vi "Set Pump Phases Parameters 2 (SubVI).vi"(0 "Units":string, 1 "Target Time":dbl, 2 "error out 2":errorcluster, 4 "Inc/Dec time":dbl, 6 "Flow rate":dbl, 7 "Previous Flow rate":dbl, 8 "Direction":string(combo), 10 "Send":bool, 11 "VISA Pump resource name out 2":refnum<visa-resource-name>) -> (3 "VISA resource name out":refnum<visa-resource-name>, 5 "error out":errorcluster)   [LabVIEW 2020]
panel:
  in  "Valve error out 2":errorcluster
  in  "Valve Position":dbl
  in  "Valve VISA resource name":refnum<visa-resource-name>
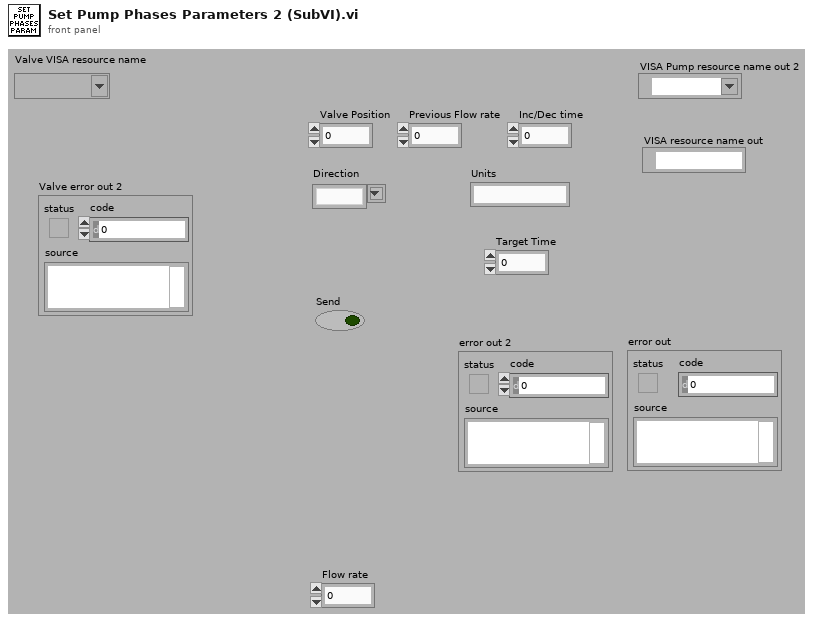
[diagram p1: front panel]
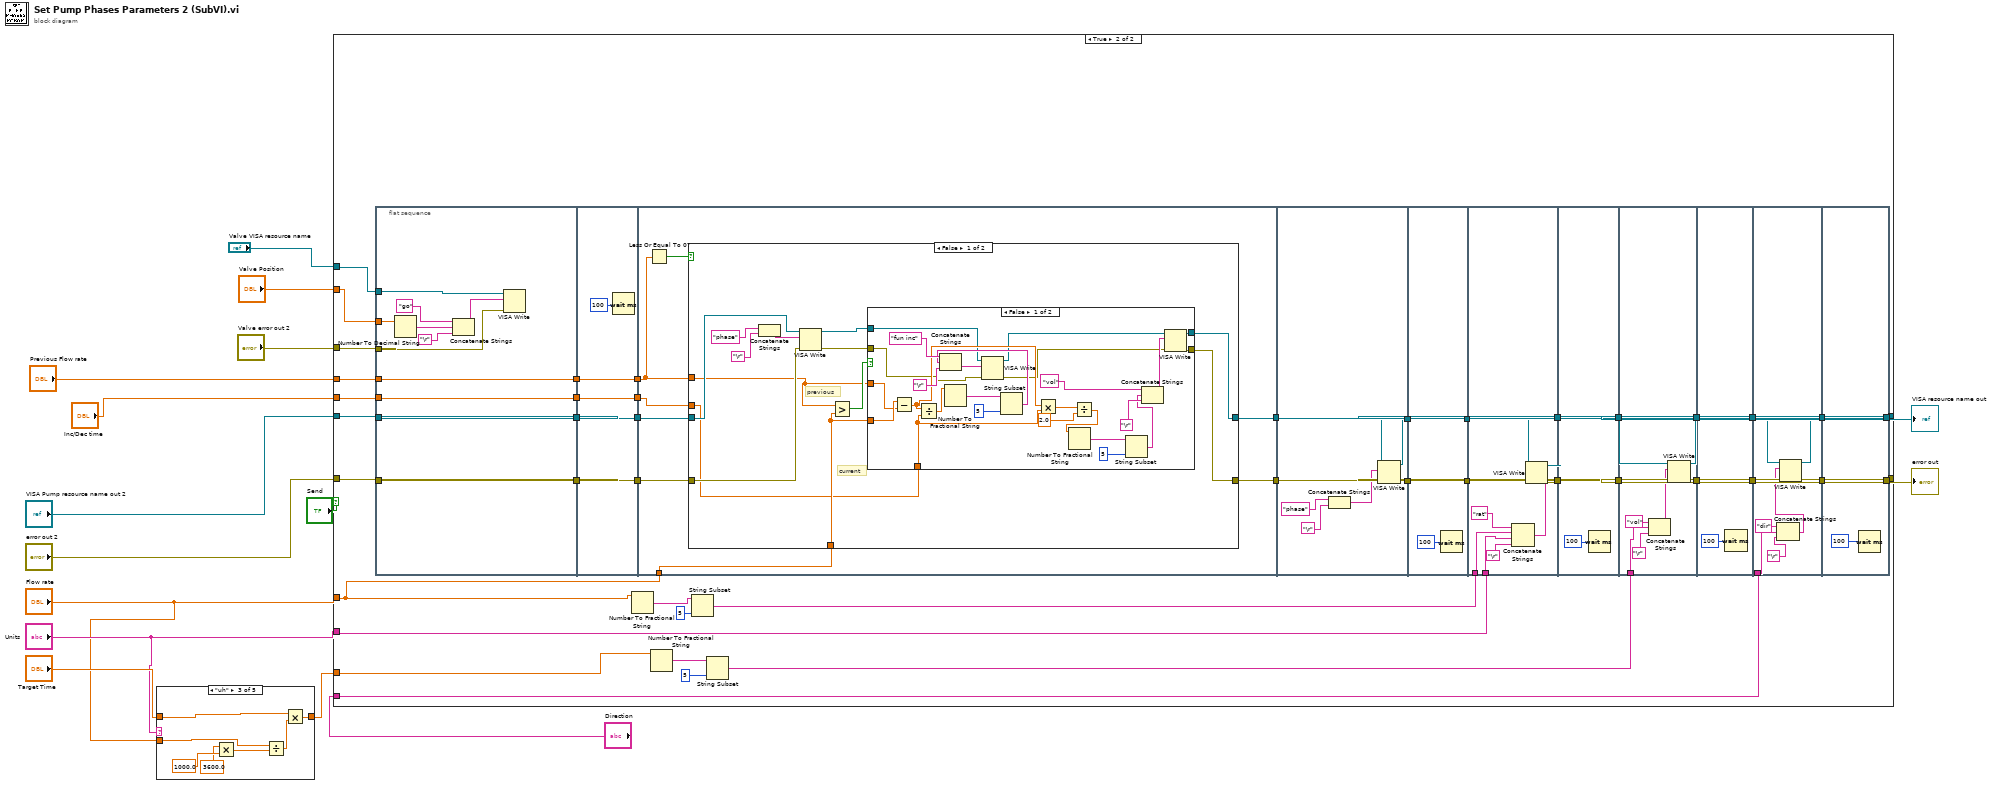
[diagram p0: block diagram]
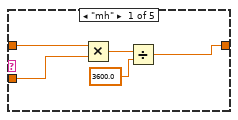
[diagram p2: hidden frame]
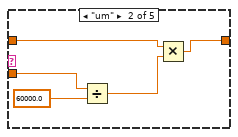
[diagram p3: hidden frame]
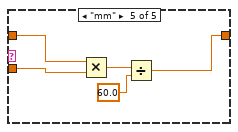
[diagram p5: hidden frame]
diagram:
  n1 = case shown="\"uh\"" "Units" {
    tunnel: "Target Time" -> [w19 w23 w29 w33 w35]
    tunnel: [w16 w24 w32 w33 w36] -> w6
    tunnel: "Flow rate" -> [w18 w25 w27 _ w34]
    frame "mh" {
      n2 = Multiply(x=w19, y=w18) -> (x*y=w20:dbl)
      n3 = Divide(x=w20, y=3600.0) -> (x/y=w16:dbl)
    }
    frame "um" {
      n4 = Divide(x=w25, y=60000.0) -> (x/y=w22:dbl)
      n5 = Multiply(x=w23, y=w22) -> (x*y=w24:dbl)
    }
    frame "uh" {
      n6 = Multiply(x=3600.0 ("y"), y=1000.0 ("x")) -> (x*y=w26:dbl)
      n7 = Divide(x=w27, y=w26) -> (x/y=w31:dbl)
      n8 = Multiply(x=w29, y=w31) -> (x*y=w32:dbl)
    }
    frame Default {
    }
    frame "mm" {
      n9 = Multiply(x=w35, y=w34) -> (x*y=w38:dbl)
      n10 = Divide(x=w38, y=60.0) -> (x/y=w36:dbl)
    }
  }
  n11 = case shown="True" "Send" {
    tunnel: "VISA Pump resource name out 2" -> [w40 w83]
    tunnel: "error out 2" -> [w39 w82]
    tunnel: [w40 w81] -> w14
    tunnel: [w39 w80] -> w15
    tunnel: "Flow rate" -> [_ w41]
    tunnel: "Units" -> [_ w79]
    tunnel: w6 -> [_ w57]
    tunnel: "Direction" -> [_ w66]
    tunnel: "Valve Position" -> [_ w55]
    tunnel: "Valve VISA resource name" -> [_ w56]
    tunnel: "Valve error out 2" -> [_ w54]
    tunnel: "Previous Flow rate" -> [_ w47]
    tunnel: "Inc/Dec time" -> [_ w43]
    frame False {
    }
    frame True {
      n12 = flat-sequence {
        tunnel: w82 -> [w93]
        tunnel: w83 -> [w94]
        tunnel: [w94] -> w53
        tunnel: [w93] -> w52
        tunnel: w56 -> [w88]
        tunnel: w55 -> [w87]
        tunnel: w54 -> [w86]
        tunnel: [w85] -> w48
        tunnel: w47 -> [w85]
        tunnel: [w84] -> w44
        tunnel: w43 -> [w84]
        tunnel: w53 -> [w99]
        tunnel: [w99] -> w51
        tunnel: w52 -> [w98]
        tunnel: [w98] -> w50
        tunnel: w48 -> [w96]
        tunnel: [w96] -> w46
        tunnel: w44 -> [w95]
        tunnel: [w95] -> w42
        tunnel: w51 -> [w106]
        tunnel: w50 -> [w104]
        tunnel: [w103] -> w49
        tunnel: w46 -> [w100]
        tunnel: [w105] -> w45
        tunnel: w42 -> [w102]
        tunnel: w41 -> [w101]
        tunnel: [w155] -> w78
        tunnel: [w154] -> w76
        tunnel: w49 -> [w156]
        tunnel: w45 -> [w157]
        tunnel: w78 -> [w160]
        tunnel: [w160] -> w77
        tunnel: w76 -> [w159]
        tunnel: [w159] -> w75
        tunnel: w77 -> [w169]
        tunnel: w75 -> [w167]
        tunnel: w62 -> [w164]
        tunnel: w79 -> [w163]
        tunnel: [w168] -> w74
        tunnel: [w166] -> w72
        tunnel: w74 -> [w172]
        tunnel: [w172] -> w73
        tunnel: w72 -> [w171]
        tunnel: [w171] -> w71
        tunnel: w73 -> [w178]
        tunnel: w71 -> [w177]
        tunnel: w58 -> [w174]
        tunnel: [w179] -> w70
        tunnel: [w180] -> w69
        tunnel: w70 -> [w183]
        tunnel: w69 -> [w182]
        tunnel: [w183] -> w68
        tunnel: [w182] -> w67
        tunnel: w68 -> [w191]
        tunnel: w67 -> [w188]
        tunnel: w66 -> [w184]
        tunnel: [w190] -> w65
        tunnel: [w189] -> w64
        tunnel: [w193] -> w80
        tunnel: [w194] -> w81
        tunnel: w65 -> [w194]
        tunnel: w64 -> [w193]
        frame #0 {
          n13 = Number To Decimal String(number=w87) -> (decimal integer string=w92:string)  [unwired: 1 in]
          n14 = Concatenate Strings("go", w92, "\r") -> (w91:string)
          n15 = VISA Write(VISA resource name=w88, write buffer=w91, error in (no error)=w86) -> ()  [unwired: 3 out]
        }
        frame #1 {
          n16 = Wait (ms)(milliseconds to wait=u32 100) -> ()  [unwired: 1 out]
        }
        frame #2 {
          n17 = Less Or Equal To 0?(x=w100) -> (x <= 0?=w107:bool)
          n18 = case shown="False" w107 {
            tunnel: [w109 w150] -> w105
            tunnel: w106 -> [w117 w150]
            tunnel: [w108 w149] -> w103
            tunnel: w104 -> [w116 w149]
            tunnel: w102 -> [w112 _]
            tunnel: w101 -> [w114 _]
            tunnel: w100 -> [w113 _]
            frame False {
              # "previous"
              # "current"
              n19 = Concatenate Strings("phase" ("string"), "\r") -> (w120:string)
              n20 = VISA Write(VISA resource name=w117, write buffer=w120, error in (no error)=w116) -> (VISA resource name out=w111:refnum<visa-resource-name>, error out=w110:errorcluster)  [unwired: 1 out]
              n21 = Greater?(x=w113, y=w114) -> (0:w115:bool)
              n22 = case shown="False" w115 {
                tunnel: w114 -> [w143 _]
                tunnel: w113 -> [w142 _]
                tunnel: w112 -> [w133 _]
                tunnel: w111 -> [w126 w148]
                tunnel: w110 -> [w125 w147]
                tunnel: [w122 w148] -> w109
                tunnel: [w121 w147] -> w108
                frame False {
                  n23 = Subtract(x=w143, y=w142) -> (x-y=w134:dbl)
                  n24 = Divide(x=w134, y=w133) -> (x/y=w139:dbl)
                  n25 = Number To Fractional String(number=w139) -> (F-format string=w141:string)  [unwired: 3 in]
                  n26 = String Subset(string=w141, length (rest)=5 ("length (rest)")) -> (substring=w138:string)  [unwired: 1 in]
                  n27 = Concatenate Strings("fun inc" ("string"), w138, "\r") -> (w146:string)
                  n28 = VISA Write(VISA resource name=w126, write buffer=w146, error in (no error)=w125) -> (VISA resource name out=w124:refnum<visa-resource-name>, error out=w123:errorcluster)  [unwired: 1 out]
                  n29 = Multiply(x=w134, y=w133) -> (x*y=w132:dbl)
                  n30 = Divide(x=w132, y=2.0) -> (x/y=w128:dbl)
                  n31 = Number To Fractional String(number=w128) -> (F-format string=w130:string)  [unwired: 3 in]
                  n32 = String Subset(string=w130, length (rest)=5 ("length (rest)")) -> (substring=w127:string)  [unwired: 1 in]
                  n33 = Concatenate Strings("vol" ("string"), w127, "\r") -> (w135:string)
                  n34 = VISA Write(VISA resource name=w124, write buffer=w135, error in (no error)=w123) -> (VISA resource name out=w122:refnum<visa-resource-name>, error out=w121:errorcluster)  [unwired: 1 out]
                }
                frame True {
                }
              }
            }
            frame True {
            }
          }
        }
        frame #3 {
          n35 = Concatenate Strings("phase" ("string"), "\r") -> (w153:string)
          n36 = VISA Write(VISA resource name=w157, write buffer=w153, error in (no error)=w156) -> (VISA resource name out=w155:refnum<visa-resource-name>, error out=w154:errorcluster)  [unwired: 1 out]
        }
        frame #4 {
          n37 = Wait (ms)(milliseconds to wait=u32 100) -> ()  [unwired: 1 out]
        }
        frame #5 {
          n38 = Concatenate Strings("rat" ("string"), w164, w163, "\r") -> (w161:string)
          n39 = VISA Write(VISA resource name=w169, write buffer=w161, error in (no error)=w167) -> (VISA resource name out=w168:refnum<visa-resource-name>, error out=w166:errorcluster)  [unwired: 1 out]
        }
        frame #6 {
          n40 = Wait (ms)(milliseconds to wait=u32 100) -> ()  [unwired: 1 out]
        }
        frame #7 {
          n41 = Concatenate Strings("vol" ("string"), w174, "\r") -> (w173:string)
          n42 = VISA Write(VISA resource name=w178, write buffer=w173, error in (no error)=w177) -> (VISA resource name out=w179:refnum<visa-resource-name>, error out=w180:errorcluster)  [unwired: 1 out]
        }
        frame #8 {
          n43 = Wait (ms)(milliseconds to wait=u32 100) -> ()  [unwired: 1 out]
        }
        frame #9 {
          n44 = Concatenate Strings("dir" ("string"), w184, "\r") -> (w187:string)
          n45 = VISA Write(VISA resource name=w191, write buffer=w187, error in (no error)=w188) -> (VISA resource name out=w190:refnum<visa-resource-name>, error out=w189:errorcluster)  [unwired: 1 out]
        }
        frame #10 {
          n46 = Wait (ms)(milliseconds to wait=u32 100) -> ()  [unwired: 1 out]
        }
      }
      n47 = Number To Fractional String(number=w41) -> (F-format string=w61:string)  [unwired: 3 in]
      n48 = Number To Fractional String(number=w57) -> (F-format string=w60:string)  [unwired: 3 in]
      n49 = String Subset(string=w61, length (rest)=5 ("length (rest)")) -> (substring=w62:string)  [unwired: 1 in]
      n50 = String Subset(string=w60, length (rest)=5 ("length (rest)")) -> (substring=w58:string)  [unwired: 1 in]
    }
  }
  "error out" <- w15
  "VISA resource name out" <- w14
